vi "Hardware-ESTTL.vi"(8 "error in (no error)":errorcluster, 11 "DCM-DSI in":refnum<class "DCM-DSI.lvclass">) -> (0 "error out":errorcluster, 3 "DCM-DSI out":refnum<class "DCM-DSI.lvclass">)   [LabVIEW 2016, in "DSI-RT.lvlib"]
uses:
  DSI-RT.lvlib
  Classes/DCM-DSI/DCM-DSI.lvclass
  Classes/DCM-DSI/Read DCM Ref.vi
  Classes/DCM-DSI/Read ESTTL Setup.vi
  Classes/DCM-DSI/Write ESTTL Setup.vi
  <vilib>/Powertrain Controls/Device Drivers/DCM/Rev0/RT/DCM - RT.lvclass
  <vilib>/Powertrain Controls/Device Drivers/DCM/ESTTL/RT/DCM - RT - ESTTL.lvlib
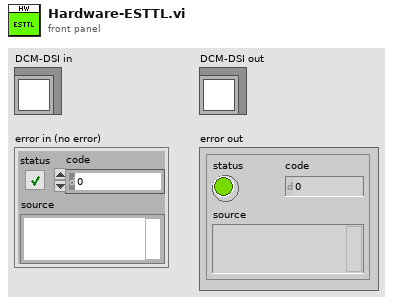
[diagram p1: front panel]
types:
  T1 = typedef "DCM - RT - ESTTL.lvlib/Setup.ctl" = cluster{"Mode":T2, "Polarity":bool, "Frequency [Hz]":sgl, "Duty Cycle [%]":sgl, "TDC Offset [CAD]":sgl, "Window Start [DBTDC]":sgl, "Window End [DBTDC]":sgl, "Angles":T3[], "Skip Fire":bool, "Skip Fire Index":u8}
  T2 = typedef "DCM - FPGA - ESTTL.lvlib/Mode.ctl" = enum8{"Off", "Pulse Width Modulation", "Engine Position Tracking"}
  T3 = typedef "DCM - RT - ESTTL.lvlib/Angle Control.ctl" = cluster{"Enable":bool, "Location [DBTDC]":sgl, "Duration [s]":sgl}
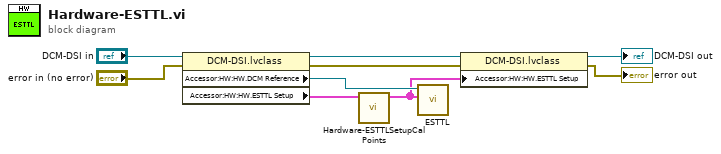
[diagram p0: block diagram]
diagram:
  n1 = property class="DCM-DSI.lvclass"(reference="DCM-DSI in", error in="error in (no error)") -> (reference out=w3:refnum<class "DCM-DSI.lvclass">, error out=w1:errorcluster, "Accessor:HW:HW.DCM Reference"=w9:refnum<class "DCM - RT.lvclass">, "Accessor:HW:HW.ESTTL Setup"=w6:T1[])
  n2 = call "Hardware-ESTTLSetupCalPoints.vi"("ESTTL Setup"=w6) -> ("ESTTL Setup"=w2:T1[])  [unwired: 10 in]
  n3 = call <vilib>:"ESTTL.vi"("ESTTL Setup"=w2, "DCM Reference"=w9) -> ()  [unwired: 10 in]
  n4 = property class="DCM-DSI.lvclass"(reference=w3, error in=w1, "Accessor:HW:HW.ESTTL Setup"=w2) -> (reference out=→"DCM-DSI out":refnum<class "DCM-DSI.lvclass">, error out=→"error out":errorcluster)
